vi "WRITE - File.vi"(0 "reference in":refnum<class "HeadAcousticHDF.lvclass">, 5 "error in (no error)":errorcluster, 7 "TDMS Path - WRITE":path) -> (14 "reference out":refnum<class "HeadAcousticHDF.lvclass">, 19 "error out":errorcluster)   [LabVIEW 2022 SP3, in "HeadAcousticHDF.lvclass"]
uses:
  HeadAcousticHDF.lvclass
  API/GSwFormDSP_class/functions/Attribute List.ctl
  <vilib>/Platform/storage/Storage.llb/usiSequenceRepresentation.ctl
  <vilib>/Platform/storage/lvStorage.llb/_openStorageWithRootAutoDetect.vi
  <vilib>/Platform/storage/lvStorage.llb/xStorage/xStorageSupp/ErrorOut.vi
  <vilib>/Platform/storage/lvStorage.llb/_createOrGetExplicitChildObject.vi
  <vilib>/Platform/storage/lvStorage.llb/_prepDDT.vi
  <vilib>/Platform/storage/lvStorage.llb/_getChannelNameFromDDT.vi
  <vilib>/Platform/storage/lvStorage.llb/_createOrGetByNameExplicitChildObject.vi
  <vilib>/Platform/storage/lvStorage.llb/_saveDDT.vi
  <vilib>/Platform/storage/Storage.llb/Get Object Info.vi
  <vilib>/Platform/storage/Storage.llb/__closeStorageFromObject.vi
  <vilib>/Platform/storage/lvStorage.llb/xStorage/Open Data Storage/Open Data Storage.xnode
  <vilib>/Platform/storage/lvStorage.llb/xStorage/Write Data/Write Data.xnode
  <vilib>/Platform/storage/lvStorage.llb/xStorage/Close Data Storage/Close Data Storage.xnode
  API/GSwFormDSP_class/GSwFormDSP.lvclass
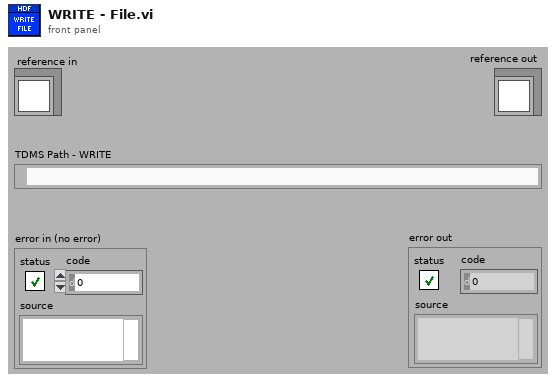
[diagram p1: front panel]
types:
  T1 = typedef "GSwFormDSP.lvclass/Attribute List.ctl" = string
  T2 = enum16{"Append values", "Replace values at index", "Replace all values"}
  T3 = enum16{"open", "open or create", "create or replace", "create", "open (read only)"}
  T4 = enum16{"UPDATE", "READ", "QUERY", "CREATE CHILD", "CREATE", "CONNECT", "DISCONNECT"}
  T5 = typedef "usiSequenceRepresentation.ctl" = enum16{"explicit", "implicit"}
  T6 = typedef "HeadAcousticHDF.lvclass/ObjectAttributes.ctl" = cluster{"Time Data":refnum<class "GSwFormDSP.lvclass">, "Data Plugin Name":string, "Additional Data Plugin Name":string, "New Time Data Obj?":bool}
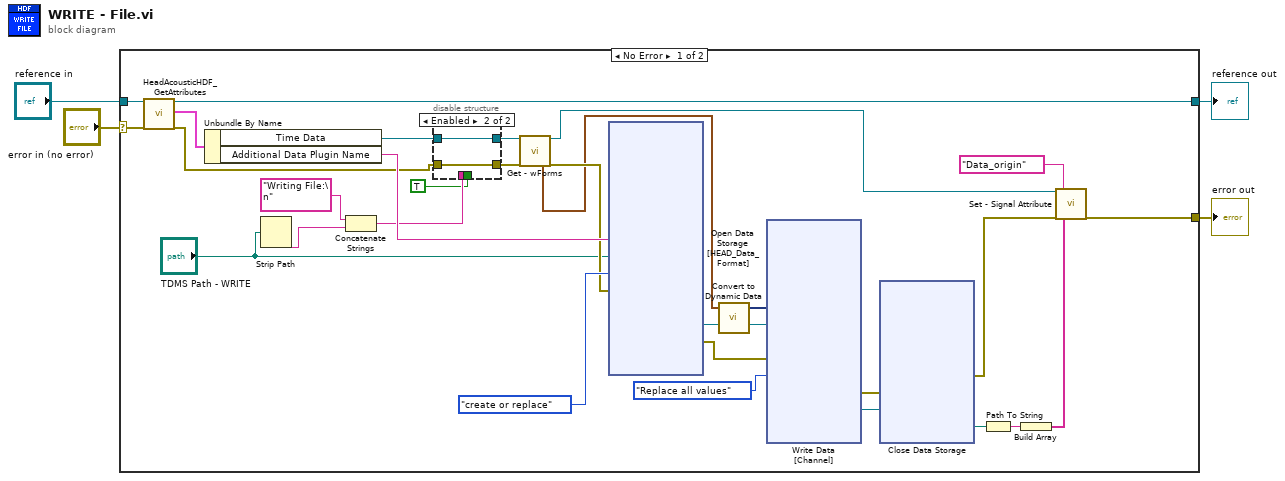
[diagram p0: block diagram]
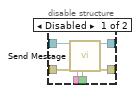
[diagram p2: hidden frame]
diagram:
  n1 = case shown="No Error" "error in (no error)" {
    selector: "error in (no error)" -> [w34 w91]
    tunnel: [w5 w91] -> w3
    tunnel: [w33 w90] -> w1
    tunnel: "reference in" -> [w31 w90]
    frame No Error {
      n2 = call "HeadAcousticHDF_GetAttributes.vi"("reference in"=w31, "error in (no error)"=w34) -> ("reference out"=w33:refnum<class "HeadAcousticHDF.lvclass">, "attributes"=w32:T6, "error out"=w14:errorcluster)  [unwired: 14 in, 1 out]
      n3 = Unbundle By Name(w32) -> ("Time Data"=w16:refnum<class "GSwFormDSP.lvclass">, "Additional Data Plugin Name"=w30:string)
      n4 = Strip Path(path="TDMS Path - WRITE") -> (name=w19:string)  [unwired: 1 out]
      n5 = Concatenate Strings("Writing File:\n", w19) -> (w18:string)
      n6 = disable-structure shown="Enabled" {
        disable-tunnel: w18 -> [w40 _]
        disable-tunnel: TRUE ("Make Cursor Busy?") -> [w39 _]
        disable-tunnel: w16 -> [w38 w42]
        disable-tunnel: [w37 w42] -> w15
        disable-tunnel: w14 -> [w36 w41]
        disable-tunnel: [w35 w41] -> w13
        frame Disabled {
          n7 = call-dynamic "Send Message.vi"("reference in"=w38, "error in (no error)"=w36, "Message (\"\" closes the window)"=w40, "Make Cursor Busy?"=w39) -> ("reference out"=w37:refnum<class "GSwFormDSP.lvclass">, "error out"=w35:errorcluster)  [unwired: 14 in]
        }
        frame Enabled {
        }
      }
      n8 = call-dynamic "Get - wForms.vi"("reference in"=w15, "error in (no error)"=w13) -> ("wForms"=w21:waveform(dbl)[], "reference out"=w10:refnum<class "GSwFormDSP.lvclass">, "error out"=w28:errorcluster)  [unwired: 14 in, 1 out]
      n9 = xnode "Open Data Storage\n[HEAD_Data_Format]"("DataPlugin name"=w30, "file path"="TDMS Path - WRITE", "function (open:0)"=T3."create or replace", "error in (no error)"=w28) -> ("storage refnum (file)"=w25:refnum<k20>, "error out"=w26:errorcluster)  [unwired: 1 in, 1 out]
      n10 = call "Convert to Dynamic Data"("Array of Waveforms"=w21) -> ("Dynamic Data Type"=w22:dynamicdata)  [unwired: 3 in]
      n11 = xnode "Write Data\n[Channel]"("Signal"=w22, "storage refnum (file)"=w25, "error in"=w26, "append / replace (append data values)"=T2."Replace all values") -> ("error out"=w23:errorcluster, "storage refnum (file) out"=w24:refnum<k20>)  [unwired: 1 in, 1 out]
      n12 = xnode "Close Data Storage\n"("error in (no error)"=w23, "storage refnum (file)"=w24) -> ("error out"=w11:errorcluster, "file path"=w8:path)
      n13 = Path To String(path=w8) -> (string=w7:string)
      n14 = Build Array(w7) -> (w6:string[])
      n15 = call-dynamic "Set - Signal Attribute.vi"("reference in"=w10, "error in (no error)"=w11, "wForm Attributes"=T1 "Data_origin", "Attribute"=w6) -> ("error out"=w5:errorcluster)  [unwired: 14 in, 1 out]
    }
    frame Error {
    }
  }
  "error out" <- w3
  "reference out" <- w1
